vi "Get VI server port from LV Version.vi"(8 "error in (no error)":errorcluster, 11 "input string":string) -> (0 "error out":errorcluster, 1 "LabVIEW path":string, 2 "appended path":path, 3 "VI Server port":u32)   [LabVIEW 2021]
uses:
  <vilib>/Utility/config.llb/Read Key (U32).vi
  <vilib>/Utility/config.llb/NI_LVConfig.lvlib
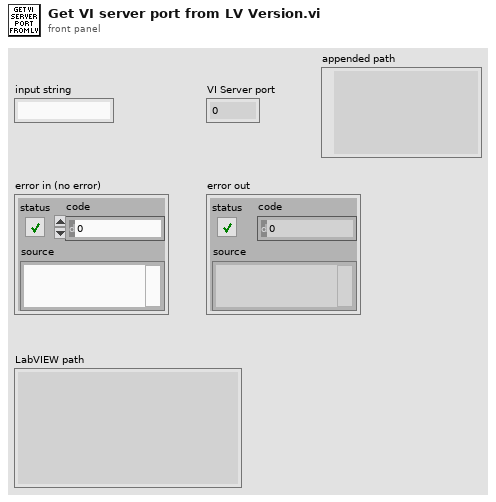
[diagram p1: front panel]
types:
  T1 = typedef "NI_LVConfig.lvlib/Config Data RefNum.ctl" = refnum<k1>
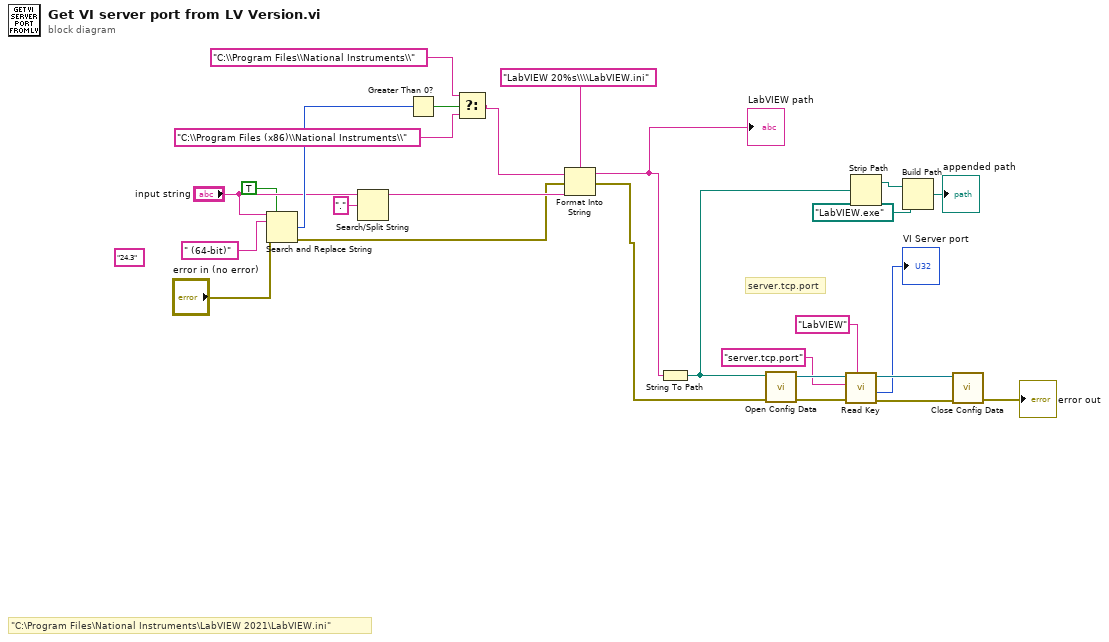
[diagram p0: block diagram]
diagram:
  (unwired) "24.3"
  # "server.tcp.port"
  # "\"C:\\Program Files\\National Instruments\\LabVIEW 2021\\LabVIEW.ini\""
  n1 = Search and Replace String(replace all?=TRUE ("replace all? (F)"), input string="input string", search string=" (64-bit)", error in="error in (no error)") -> (number of replacements=w26:i32, error out=w19:errorcluster)  [unwired: 4 in, 2 out]
  n2 = Search/Split String(string="input string", search string/char (-)=".") -> (substring before match=w21:string)  [unwired: 1 in, 2 out]
  n3 = Greater Than 0?(x=w26) -> (x > 0?=w25:bool)
  n4 = Select(t="C:\\Program Files\\National Instruments\\" ("input string"), s=w25, f="C:\\Program Files (x86)\\National Instruments\\" ("input string")) -> (s? t:f=w17:string)
  n5 = Format Into String(format string="LabVIEW 20%s\\\\LabVIEW.ini", initial string=w17, error in=w19, w21) -> (resulting string=w7:string, error out=w13:errorcluster)
  "LabVIEW path" <- w7
  n6 = String To Path(string=w7) -> (path=w4:path)
  n7 = call <vilib>:"Open Config Data.vi"("error in (no error)"=w13, "configuration file path"=w4) -> ("error out"=w15:errorcluster, "refnum"=w14:T1)  [unwired: 7 in, 1 out]
  n8 = call-poly <vilib>:"Read Key.vi"("section"="LabVIEW", "error in (no error)"=w15, "key"="server.tcp.port" ("section"), "refnum"=w14) -> ("error out"=w10:errorcluster, "value"=→"VI Server port":u32, "refnum out"=w9:T1)  [unwired: 4 in, 1 out]
  n9 = Strip Path(path=w4) -> (stripped path=w3:path)  [unwired: 1 out]
  n10 = Build Path(base path=w3, name or relative path=path "LabVIEW.exe") -> (appended path=→"appended path":path)
  n11 = call <vilib>:"Close Config Data.vi"("error in (no error)"=w10, "refnum"=w9) -> ("error out"=→"error out":errorcluster)  [unwired: 8 in, 1 out]
